vi "11 Execution Order.vi"() -> ()   [LabVIEW 2020]
uses:
  _Subs/OpenDiagram/Open_XControl.xctl
panel:
  in  "OpenDiag":refnum<vi>(xcontrol)
  out "Counter 6":i32
  out "Counter 5":i32
  out "Counter 3":i32
  out "Counter 4":i32
  out "Counter 2":i32
  out "Counter 1":i32
  # "11 Execution Order\nThis code shows how things can run simultaniously (in parallel) or sequentially\n\nInstructions:\n1. Hit the Run arrow and see the numbers change\n2. Try running with execution highlighting (lightbulb) on."
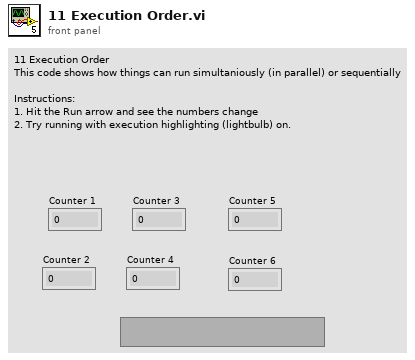
[diagram p1: front panel]
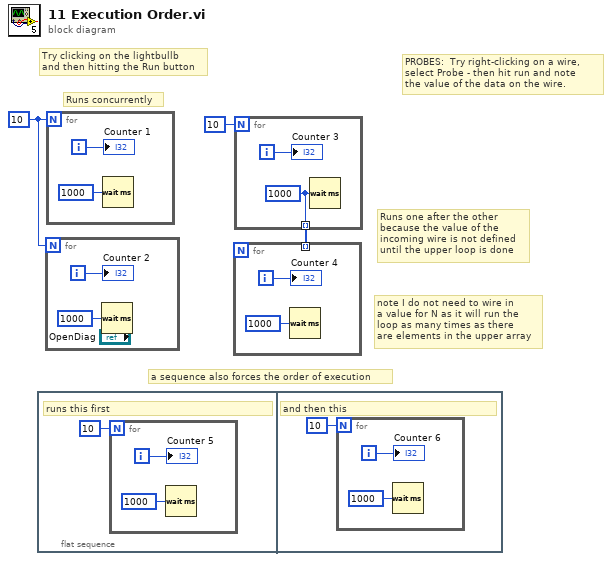
[diagram p0: block diagram]
diagram:
  w3 = 10
  # "PROBES:  Try right-clicking on a wire,\nselect Probe - then hit run and note\nthe value of the data on the wire."
  # "note I do not need to wire in\na value for N as it will run the \nloop as many times as there\nare elements in the upper array"
  # "a sequence also forces the order of execution"
  # "Runs one after the other\nbecause the value of the\nincoming wire is not defined\nuntil the upper loop is done"
  # "Runs concurrently"
  # "Try clicking on the lightbullb\nand then hitting the Run button"
  n1 = flat-sequence {
    frame #0 {
      # "runs this first"
      n2 = for {
        N: 10 -> [_]
        i -> [w6]
        n3 = Wait (ms)(milliseconds to wait=u32 1000) -> ()  [unwired: 1 out]
        "Counter 5" <- w6
      }
    }
    frame #1 {
      # "and then this"
      n4 = for {
        N: 10 -> [_]
        i -> [w9]
        n5 = Wait (ms)(milliseconds to wait=u32 1000) -> ()  [unwired: 1 out]
        "Counter 6" <- w9
      }
    }
  }
  n6 = for {
    N: w3 -> [_]
    i -> [w11]
    n7 = Wait (ms)(milliseconds to wait=u32 1000) -> ()  [unwired: 1 out]
    "Counter 2" <- w11
  }
  n8 = for {
    N: w3 -> [_]
    i -> [w13]
    n9 = Wait (ms)(milliseconds to wait=u32 1000) -> ()  [unwired: 1 out]
    "Counter 1" <- w13
  }
  n10 = for {
    N: 10 -> [_]
    tunnel: [w14] -> w1 mode=indexing
    i -> [w15]
    w14 = u32 1000 ("milliseconds to wait")
    n11 = Wait (ms)(milliseconds to wait=w14) -> ()  [unwired: 1 out]
    "Counter 3" <- w15
  }
  n12 = for {
    tunnel: w1 -> [_] mode=indexing
    i -> [w17]
    n13 = Wait (ms)(milliseconds to wait=u32 1000) -> ()  [unwired: 1 out]
    "Counter 4" <- w17
  }
